vi "EXAMPLE Fetch Query.vi"(8 "error in (no error)":errorcluster, 11 "VISA resource name":refnum<visa-resource-name>) -> (0 "error out":errorcluster, 2 "Result":string, 3 "VISA resource name out":refnum<visa-resource-name>)   [LabVIEW 2025]
doc: "Chroma\n5 Clock Tower Place Suite 210\nMaynard, MA 01754\nTel: 1 800 253-1230\nTel: 1 877 4 A HIPOT\nFax: 1 978-461-4295\nWebsite: www.chroma.com"
uses:
  <instrlib>/Chroma 19052/Chroma 19052.lvlib
panel:
  # "Example"
  # "FETCH?"
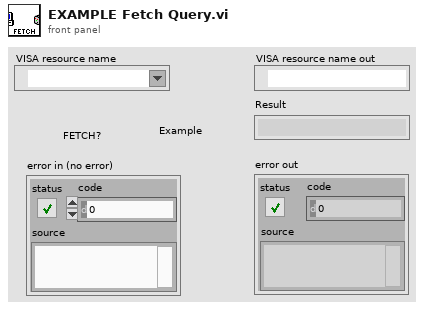
[diagram p1: front panel]
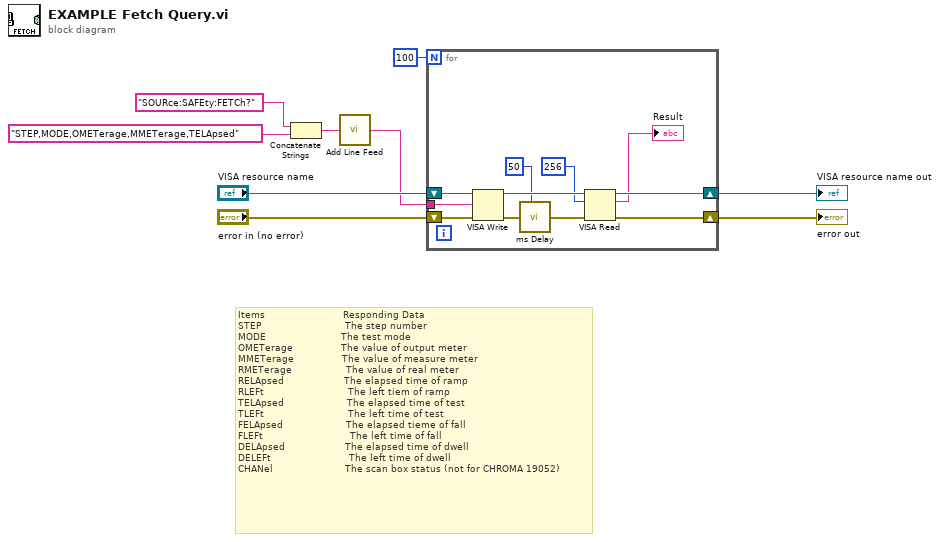
[diagram p0: block diagram]
diagram:
  # "Items                          Responding Data\nSTEP                            The step number\nMODE                         The test mode\nOMETerage                The value of output meter\nMMETerage                The value of measure meter\nRMETerage                  The value of real meter\nRELApsed                    The elapsed time of ramp \nRLEFt                            The left tiem of ramp\nTELApsed                     The elapsed time of test\nTLEFt                            The left time of test\nFELApsed                     The elapsed tieme of fall\nFLEFt                             The left time of fall\nDELApsed                    The elapsed time of dwell\nDELEFt                          The left time of dwell\nCHANel                        The scan box status (not for CHROMA 19052)"
  n1 = Concatenate Strings("SOURce:SAFEty:FETCh?", "STEP,MODE,OMETerage,MMETerage,TELApsed") -> (w2:string)
  n2 = call <instrlib>:"Add Line Feed.vi"("Command string"=w2) -> ("Concatenated string"=w7:string)  [unwired: 4 in]
  n3 = for {
    N: 100 -> [_]
    tunnel: w7 -> [w16]
    shift-right: [w14] -> w5
    shift-left: "error in (no error)" -> [w18]
    shift-right: [w15] -> w6
    shift-left: "VISA resource name" -> [w17]
    n4 = VISA Write(VISA resource name=w17, write buffer=w16, error in (no error)=w18) -> (VISA resource name out=w20:refnum<visa-resource-name>, error out=w11:errorcluster)  [unwired: 1 out]
    n5 = call <instrlib>:"ms Delay.vi"("miliseconds to wait"=u32 50 ("Time Delay ms"), "error in (no error)"=w11) -> ("error out"=w12:errorcluster)  [unwired: 6 in, 1 out]
    n6 = VISA Read(VISA resource name=w20, byte count=u32 256, error in (no error)=w12) -> (VISA resource name out=w15:refnum<visa-resource-name>, read buffer=→"Result":string, error out=w14:errorcluster)  [unwired: 1 out]
  }
  "error out" <- w5
  "VISA resource name out" <- w6
